vi "stitchingModeWeightedAverage.vi"(9 "Data In":dbl[][][](array[numeric])) -> (2 "Stitched Data Out":dbl[][](array[numeric]))   [LabVIEW 2020, in "horiba.lvlib" / "CCD.lvclass"]
doc: "Stitches spectra based on simple cut-off modus."
uses:
  CCD.lvclass
  dcc24e37-a298-45d9-8a8e-aa769f88db0e.vi
  <vilib>/Array/Sort 2D Array - Pop Stack.vi
  <vilib>/Array/Sort 2D Array - Push Stack.vi
  dcc24e37-a298-45d9-8a8e-aa769f88db0e.vi/269d4b3b-47f5-49e3-8884-44851e4dd9d5.vi
  dcc24e37-a298-45d9-8a8e-aa769f88db0e.vi/6d99389c-673d-4efb-bf33-19b32bcf4cf8.vi
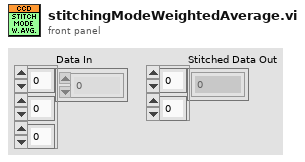
[diagram p1: front panel]
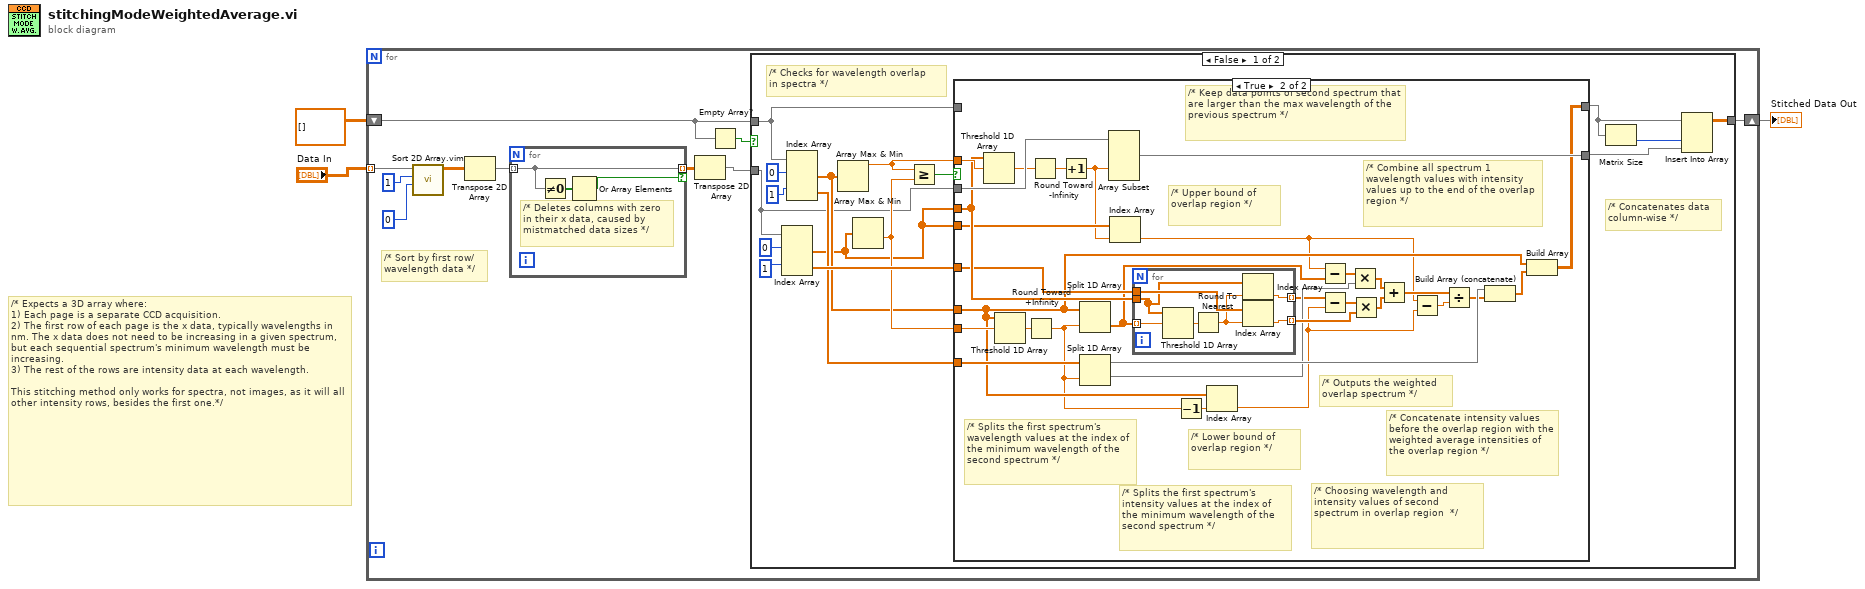
[diagram p0: block diagram]
diagram:
  # "/* Expects a 3D array where:\n1) Each page is a separate CCD acquisition.\n2) The first row of each page is the x data, typically wavelengths in nm. The x data does not need to be increasing in a given spectrum, but each sequential spectrum's minimum wavelength must be increasing.\n3) The rest of the rows are intensity data at each wavelength. \n\nThis stitching method only works for spectra, not images, as it will all other intensity rows, besides the first one.*/"
  n1 = for {
    tunnel: "Data In" -> [w7] mode=indexing
    shift-right: [w13] -> w2
    shift-left: dbl[][] [] ("Empty Array") -> [w4]
    # "/* Sort by first row/ \nwavelength data */"
    n2 = call "Sort 2D Array.vim"("index"=0, "dimension to index (column)"=1 ("index"), "2D array"=w7) -> ("sorted 2D array"=w5:dbl[][])  [unwired: 7 in, 1 out]
    n3 = Transpose 2D Array(2D array=w5) -> (transposed array=w11:dbl[][])
    n4 = for {
      tunnel: w11 -> [w15] mode=indexing
      tunnel: [w15] -> w10 mode=indexing if=w16
      # "/* Deletes columns with zero\nin their x data, caused by\nmistmatched data sizes */"
      n5 = Not Equal To 0?(x=w15) -> (x != 0?=w14:bool[])
      n6 = Or Array Elements(Boolean array=w14) -> (logical OR=w16:bool)
    }
    n7 = Transpose 2D Array(2D array=w10) -> (transposed array=w6:dbl[][])
    n8 = Empty Array?(array=w4) -> (empty?=w12:bool)
    n9 = case shown="False" w12 {
      tunnel: [w27 w74] -> w13
      tunnel: w6 -> [w18 w74]
      tunnel: w4 -> [w21 _]
      frame False {
        # "/* Concatenates data \ncolumn-wise */"
        # "/* Checks for wavelength overlap \nin spectra */"
        n10 = Index Array(array=w18, index (row) #1=0 ("index (row)"), index (row) #2=1 ("index (row)")) -> (element #1=w17:dbl[], element #2=w24:dbl[])  [unwired: 2 in]
        n11 = Index Array(array=w21, index (row) #1=0 ("index (row)"), index (row) #2=1 ("index (row)")) -> (element #1=w22:dbl[], element #2=w19:dbl[])  [unwired: 2 in]
        n12 = Array Max & Min(array=w22) -> (max value=w29:dbl)  [unwired: 3 out]
        n13 = Array Max & Min(array=w17) -> (min value=w23:dbl)  [unwired: 3 out]
        n14 = Greater Or Equal?(x=w29, y=w23) -> (x >= y?=w28:bool)
        n15 = case shown="True" w28 {
          tunnel: w18 -> [w34 w66]
          tunnel: [w34 w65] -> w30
          tunnel: w17 -> [_ w61]
          tunnel: w29 -> [_ w64]
          tunnel: w24 -> [_ w60]
          tunnel: w23 -> [_ w59]
          tunnel: w22 -> [_ w45]
          tunnel: w21 -> [w35 _]
          tunnel: [w35 w38] -> w20
          tunnel: w19 -> [_ w46]
          tunnel: w17 -> [_ w42]
          frame False {
            # "/* Passes new data unmodified if \nthere is no overlap */"
          }
          frame True {
            # "/* Splits the first spectrum's intensity values at the index of the minimum wavelength of the second spectrum */"
            # "/* Choosing wavelength and intensity values of second spectrum in overlap region  */"
            # "/* Lower bound of\noverlap region */"
            # "/* Upper bound of\noverlap region */"
            # "/* Splits the first spectrum's wavelength values at the index of the minimum wavelength of the second spectrum */"
            # "/* Outputs the weighted \noverlap spectrum */"
            # "/* Combine all spectrum 1 wavelength values with intensity values up to the end of the overlap region */"
            # "/* Concatenate intensity values before the overlap region with the weighted average intensities of the overlap region */"
            # "/* Keep data points of second spectrum that are larger than the max wavelength of the previous spectrum */"
            n16 = Threshold 1D Array(2:w64, 3:w61) -> (0:w62:dbl)  [unwired: 1 in]
            n17 = Threshold 1D Array(2:w59, 3:w45) -> (0:w47:dbl)  [unwired: 1 in]
            n18 = Round Toward +Infinity(x=w47) -> (ceil(x): smallest int >= x=w37:dbl)
            n19 = Round Toward -Infinity(1:w62) -> (0:w63:dbl)
            n20 = Increment(x=w63) -> (x+1=w41:dbl)
            n21 = Split 1D Array(array=w45, index=w37) -> (second subarray=w39:dbl[])  [unwired: 1 out]
            n22 = Split 1D Array(array=w46, index=w37) -> (first subarray=w58:dbl[], second subarray=w48:dbl[])
            n23 = Array Subset(array=w66, index (col)=w41) -> (w65:dbl[][])  [unwired: 3 in]
            n24 = Index Array(array=w42, index=w41) -> (element=w40:dbl)
            n25 = for {
              tunnel: w61 -> [w68]
              tunnel: w60 -> [w72]
              tunnel: w39 -> [w71] mode=indexing
              tunnel: [w70] -> w49 mode=indexing
              tunnel: [w67] -> w43 mode=indexing
              n26 = Threshold 1D Array(2:w71, 3:w68) -> (0:w73:dbl)  [unwired: 1 in]
              n27 = Round To Nearest(number=w73) -> (nearest integer value=w69:dbl)
              n28 = Index Array(array=w68, index=w69) -> (element=w67:dbl)
              n29 = Index Array(array=w72, index=w69) -> (element=w70:dbl)
            }
            n30 = Decrement(x=w37) -> (x-1=w44:dbl)
            n31 = Index Array(array=w45, index=w44) -> (element=w36:dbl)
            n32 = Subtract(x=w40, y=w39) -> (x-y=w56:dbl[])
            n33 = Subtract(x=w43, y=w36) -> (x-y=w55:dbl[])
            n34 = Multiply(x=w56, y=w48) -> (x*y=w54:dbl[])
            n35 = Multiply(x=w55, y=w49) -> (x*y=w53:dbl[])
            n36 = Add(x=w54, y=w53) -> (x+y=w51:dbl[])
            n37 = Subtract(x=w40, y=w36) -> (x-y=w52:dbl)
            n38 = Divide(x=w51, y=w52) -> (x/y=w50:dbl[])
            n39 = Build Array (concatenate)(w58, w50) -> (w57:dbl[])
            n40 = Build Array(w45, w57) -> (w38:dbl[][])
          }
        }
        n41 = Matrix Size(0:w20) -> (2:w31:i32)  [unwired: 1 out]
        n42 = Insert Into Array(array=w20, index (col)=w31, new element=w30) -> (w27:dbl[][])  [unwired: 1 in]
      }
      frame True {
        # "/* This case will run on the first loop iteration */"
      }
    }
  }
  "Stitched Data Out" <- w2
